vi "Initialize.vi"(8 "error in":errorcluster, 11 "Plugin in":refnum<class "FFT.lvclass">) -> (0 "error out":errorcluster, 3 "Plugin out":refnum<class "FFT.lvclass">)   [LabVIEW 2024, in "FFT.lvlib" / "FFT.lvclass"]
uses:
  FFT.lvclass
  C:/Program Files/National Instruments/LabVIEW 2024/vi.lib/FlexLogger/SDK/PluginSDK.lvlibp/PEFClasses/SDK/Plugin/Plugin.lvclass
  <vilib>/FlexLogger/SDK/PluginSDK.lvlibp/PEFClasses/SDK/System Interface/Resampling Mode.ctl
  <vilib>/FlexLogger/SDK/PluginSDK.lvlibp/PEFClasses/SDK/Processing Element/Timing Parameters.ctl
  <vilib>/FlexLogger/SDK/PluginSDK.lvlibp/PEFClasses/SDK/Processing Element/Timing Method.ctl
  <vilib>/FlexLogger/SDK/PluginSDK.lvlibp/PEFClasses/SDK/Channel/Data Type_v2.ctl
  <vilib>/FlexLogger/SDK/PluginSDK.lvlibp/PEFClasses/SDK/Producer Channel/Producer Channel.lvclass
  C:/Program Files/National Instruments/LabVIEW 2024/vi.lib/FlexLogger/SDK/PluginSDK.lvlibp/PEFClasses/SDK/Channel/Channel.lvclass
  FFT Globals.vi
  <vilib>/FlexLogger/SDK/PluginSDK.lvlibp/PEFClasses/SDK/Plugin/ParameterAccess/Write Single Channel.vi
  <vilib>/FlexLogger/SDK/PluginSDK.lvlibp/PEFClasses/SDK/Plugin/ParameterAccess/Write Boolean.vi
  <vilib>/FlexLogger/SDK/PluginSDK.lvlibp/PEFClasses/SDK/Plugin/ParameterAccess/Write I32.vi
  <vilib>/FlexLogger/SDK/PluginSDK.lvlibp/PEFClasses/SDK/Producer Channel/Create Producer Channel_v2.vi
  <vilib>/FlexLogger/SDK/PluginSDK.lvlibp/PEFClasses/SDK/Plugin/Plugin.lvclass
  <vilib>/FlexLogger/SDK/PluginSDK.lvlibp/PEFClasses/SDK/System Interface/System Interface.lvclass
  <vilib>/FlexLogger/SDK/PluginSDK.lvlibp/PEFClasses/SDK/Processing Element/Processing Element.lvclass
  <vilib>/FlexLogger/SDK/PluginSDK.lvlibp/PEFClasses/SDK/Channel/Channel.lvclass
  <vilib>/FlexLogger/SDK/PluginSDK.lvlibp
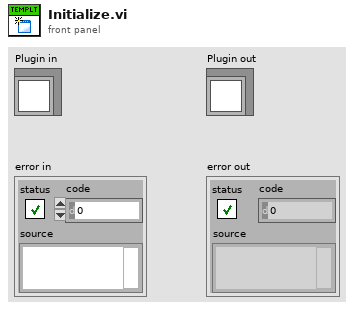
[diagram p1: front panel]
types:
  T1 = typedef "PluginSDK.lvlibp/Channel.lvclass/Data Type_v2.ctl" = u16
  T2 = typedef "PluginSDK.lvlibp/Processing Element.lvclass/Timing Parameters.ctl" = cluster{"Timing Method":T3, "Timing Period (ms)":i32}
  T3 = typedef "PluginSDK.lvlibp/Processing Element.lvclass/Timing Method.ctl" = enum16{"Periodic", "Immediate", "On Data Ready", "Triggered"}
  T4 = typedef "PluginSDK.lvlibp/System Interface.lvclass/Resampling Mode.ctl" = enum16{"No Resampling", "Custom Rate", "Maximum Rate", "Minimum Rate"}
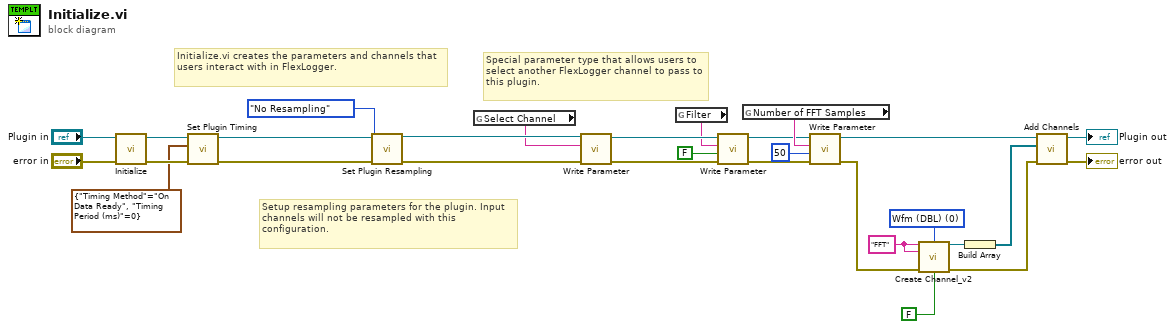
[diagram p0: block diagram]
diagram:
  w16 = "FFT" ("Unique Channel Identifier")
  w19 = T1 0 items=["Wfm (DBL)", "Wfm (Digital)", "String"] ("Data Type")
  # "Setup resampling parameters for the plugin. Input channels will not be resampled with this configuration."
  # "Special parameter type that allows users to select another FlexLogger channel to pass to this plugin."
  # "Initialize.vi creates the parameters and channels that users interact with in FlexLogger."
  n1 = call-parent "Initialize.vi"("error in (no error)"="error in", "Plugin in"="Plugin in") -> ("error out"=w22:errorcluster, "Plugin out"=w24:refnum<class "FFT.lvclass">)  [unwired: 8 in]
  n2 = call <vilib>:"Set Plugin Timing.vi"("error in (no error)"=w22, "Timing Parameters"=T2 {"Timing Method"=enum."On Data Ready", "Timing Period (ms)"=0}, "Plugin in"=w24) -> ("error out"=w21:errorcluster, "Plugin out"=w23:refnum<class "FFT.lvclass">)  [unwired: 7 in]
  n3 = call <vilib>:"Set Plugin Resampling.vi"("Plugin in"=w23, "Resampling Mode"=Resampling_Mode."No Resampling", "error in (no error)"=w21) -> ("Plugin out"=w27:refnum<class "FFT.lvclass">, "error out"=w17:errorcluster)  [unwired: 11 in]
  n4 = global read "FFT Globals.vi" "Select Channel"() -> (w25:string)
  n5 = call-poly <vilib>:"Write Parameter.vi"("error in (no error)"=w17, "Name (Unique Channel Identifier)"=w25, "Plugin in"=w27) -> ("error out"=w9:errorcluster, "Plugin out"=w12:refnum<class "FFT.lvclass">)  [unwired: 7 in]
  n6 = global read "FFT Globals.vi" "Filter"() -> (w11:string)
  n7 = call-poly <vilib>:"Write Parameter.vi"("error in (no error)"=w9, "Value"=FALSE, "Name"=w11, "Plugin in"=w12) -> ("error out"=w6:errorcluster, "Plugin out"=w7:refnum<class "FFT.lvclass">)  [unwired: 6 in]
  n8 = global read "FFT Globals.vi" "Number of FFT Samples"() -> (w8:string)
  n9 = call-poly <vilib>:"Write Parameter.vi"("error in (no error)"=w6, "Value"=50, "Name"=w8, "Plugin in"=w7) -> ("error out"=w4:errorcluster, "Plugin out"=w1:refnum<class "FFT.lvclass">)  [unwired: 6 in]
  n10 = call-poly <vilib>:"Create Channel_v2.vi"("Unique Channel Identifier"=w16, "Data Type"=w19, "Default Channel Name"=w16, "error in (no error)"=w4, "Can Disable?"=FALSE) -> ("Producer Channel"=w3:refnum<class "Producer Channel.lvclass">, "error out"=w2:errorcluster)  [unwired: 9 in]
  n11 = Build Array(w3) -> (w15:refnum<class "Producer Channel.lvclass">[])
  n12 = call <vilib>:"Add Channels.vi"("error in (no error)"=w2, "Channels"=w15, "Plugin in"=w1) -> ("error out"=→"error out":errorcluster, "Plugin out"=→"Plugin out":refnum<class "FFT.lvclass">)  [unwired: 7 in]
